vi "IFStatementParse.vi"(0 "Params":cluster{"Constant":string, "value":string}[](array[cluster]), 3 "BotSpeak in":string, 4 "Command":string, 5 "Contents":string) -> (2 "BotSpeak out":string)   [LabVIEW 2012]
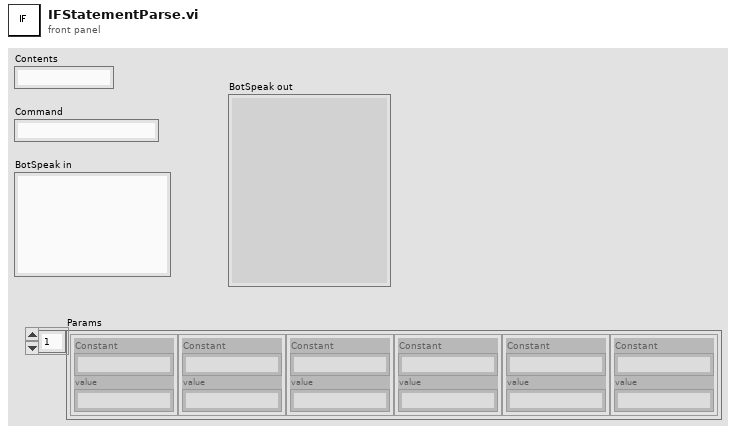
[diagram p1: front panel]
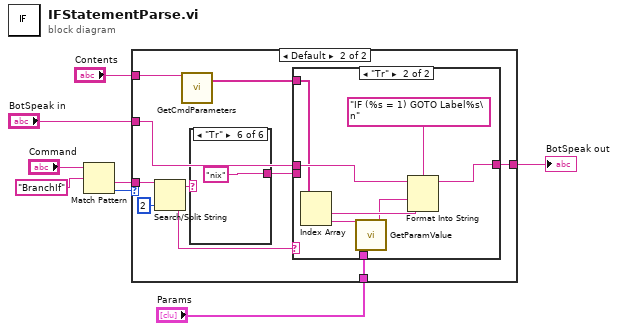
[diagram p0: block diagram]
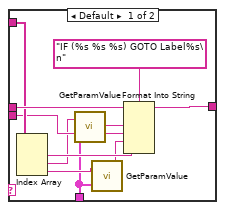
[diagram p3: hidden frame]
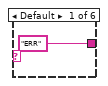
[diagram p4: hidden frame]
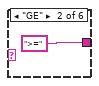
[diagram p5: hidden frame]
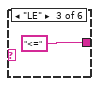
[diagram p6: hidden frame]
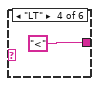
[diagram p7: hidden frame]
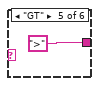
[diagram p8: hidden frame]
diagram:
  n1 = Match Pattern(string="Command", regular expression="BranchIf") -> (after substring=w6:string, offset past match=w5:i32)  [unwired: 1 in, 2 out]
  n2 = case shown="Default" w5 {
    tunnel: "BotSpeak in" -> [w9 w18]
    tunnel: [w9 w17] -> w3
    tunnel: w6 -> [_ w14]
    tunnel: "Contents" -> [_ w15]
    tunnel: "Params" -> [_ w10]
    frame -1 {
    }
    frame Default {
      n3 = Search/Split String(string=w14, offset (0)=2) -> (substring before match=w11:string)  [unwired: 1 in, 2 out]
      n4 = call "GetCmdParameters.vi"("Contents"=w15) -> ("variables"=w16:string[])  [unwired: 2 in]
      n5 = case shown="\"Tr\"" w11 {
        tunnel: ["ERR" ("regular expression") ">=" ("regular expression") "<=" ("regular expression") "<" ("regular expression") ">" ("regular expression") "nix" ("regular expression")] -> w12
        frame Default {
        }
        frame "GE" {
        }
        frame "LE" {
        }
        frame "LT" {
        }
        frame "GT" {
        }
        frame "Tr" {
        }
      }
      n6 = case shown="\"Tr\"" w11 {
        tunnel: w18 -> [w29 w37]
        tunnel: [w28 w36] -> w17
        tunnel: w16 -> [w26 w34]
        tunnel: w12 -> [w24 _]
        tunnel: w10 -> [w19 w30]
        frame Default {
          n7 = Index Array(array=w26) -> (element #1=w25:string, element #2=w21:string, element #3=w23:string)  [unwired: 3 in]
          n8 = call "GetParamValue.vi"("Params"=w19, "command"=w21) -> ("value"=w20:string)  [unwired: 1 in]
          n9 = call "GetParamValue.vi"("Params"=w19, "command"=w23) -> ("value"=w22:string)  [unwired: 1 in]
          n10 = Format Into String(format string="IF (%s %s %s) GOTO Label%s\n", initial string=w29, w20, w24, w22, w25) -> (resulting string=w28:string)  [unwired: 1 in, 1 out]
        }
        frame "Tr" {
          n11 = Index Array(array=w34) -> (element #1=w33:string, element #2=w32:string)  [unwired: 2 in]
          n12 = call "GetParamValue.vi"("Params"=w30, "command"=w32) -> ("value"=w31:string)  [unwired: 1 in]
          n13 = Format Into String(format string="IF (%s = 1) GOTO Label%s\n", initial string=w37, w31, w33) -> (resulting string=w36:string)  [unwired: 1 in, 1 out]
        }
      }
    }
  }
  "BotSpeak out" <- w3
